vi "check_visa_support.vi"(8 "error in":errorcluster) -> (0 "error out":errorcluster, 3 "visa supported":bool)   [LabVIEW 2020]
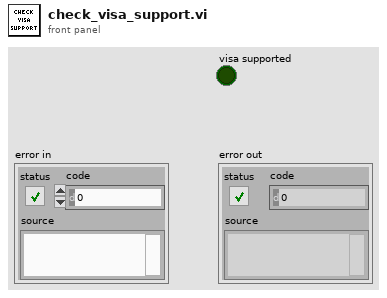
[diagram p1: front panel]
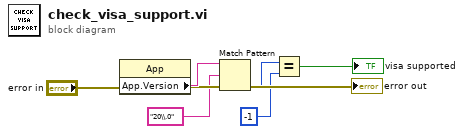
[diagram p0: block diagram]
diagram:
  n1 = property class="App"(error in="error in") -> (error out=→"error out":errorcluster, "App.Version"=w7:string)  [unwired: 1 in, 1 out]
  n2 = Match Pattern(string=w7, regular expression="20\\.0") -> (offset past match=w3:i32)  [unwired: 1 in, 3 out]
  n3 = Equal?(x=w3, y=-1) -> (x = y?=→"visa supported":bool)
